vi "Actor Core.vi"(8 "error in":errorcluster, 11 "Test Executive Builder Active Version View In":refnum<class "Test Executive Builder Active Version View.lvclass">) -> (0 "error out":errorcluster, 3 "Actor out":refnum<class "Actor.lvclass">)   [LabVIEW 2017, in "Test Executive Builder Active Version View.lvclass"]
doc: "(<B>Filename</B>: Actor Framework.lvlib:Actor.lvclass:Actor Core.vi)\n\nReceives messages to the actor, reacts to them, and initiates any error handling that may shut the actor down.\n\nDescendant classes may override this VI to append parallel tasks for the actor to complete while it handles messages. Overrides use the Call Parent Method node.\n\n<License>\nCopyright © 2017 Composed Systems, LLC | All rights reserved\nwww.composed.io\n\nAuthor: Ethan Stern <ethan.stern@composed.io>\n\nThis software is provided \"AS IS\" WITHOUT WARRANTIES, either express or implied, AND IS FOR EDUCATIONAL PURPOSES ONLY.\n</License>"
uses:
  Test Executive Builder Active Version View.lvclass
  <vilib>/gpm_packages/@cs/mva-viewable/Source/IViewable/IViewable/IViewable.lvclass
  C:/Users/jonmc/Documents/Git/Test Executive Builder/gpm_packages/@cs/mva-viewable/Source/IViewable/IViewable/IViewable.lvclass
  <vilib>/ActorFramework/Actor/Actor.lvclass
panel:
  out "Active Test Version":string
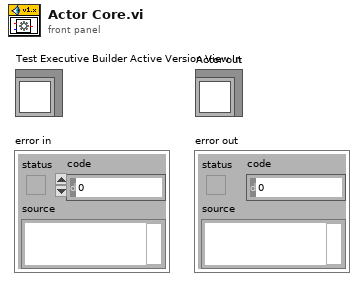
[diagram p1: front panel]
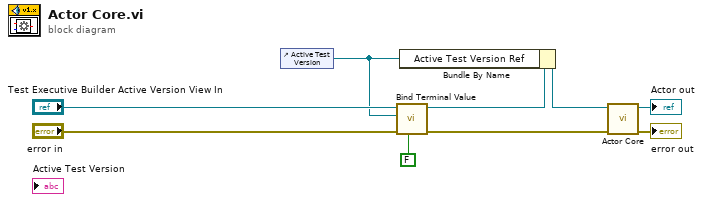
[diagram p0: block diagram]
diagram:
  n1 = control-ref of="Active Test Version"() -> (w1:refnum<vi>)
  n2 = call <vilib>:"Bind Terminal Value.vi"("Value Changes Only? (T)"=FALSE, "error in (no error)"="error in", "Ctl Refnum"=w1, "IViewable in"="Test Executive Builder Active Version View In") -> ("error out"=w5:errorcluster, "IViewable out"=w3:refnum<class "Test Executive Builder Active Version View.lvclass">)  [unwired: 6 in]
  n3 = Bundle By Name(cluster=w3, "Active Test Version Ref"=w1) -> (w2:refnum<class "Test Executive Builder Active Version View.lvclass">)
  n4 = call-parent "Actor Core.vi"("error in"=w5, "IViewable In"=w2) -> ("error out"=→"error out":errorcluster, "Actor out"=→"Actor out":refnum<class "Actor.lvclass">)  [unwired: 8 in]
